vi "Queue Byte.vi"(8 "error in":errorcluster, 10 "byte":u8 format="%02x", 11 "Buffer":refnum<data-value>) -> (0 "error out":errorcluster, 1 "overflowed?":bool, 2 "overflow":u8 format="%02x", 3 "Buffer":refnum<data-value>)   [LabVIEW 2013, in "CircularBuffer.lvlib" / "ByteFIFO.lvclass"]
doc: "This VI writes one data element into the current location in the buffer. The location in the buffer is updated automatically."
uses:
  ByteFIFO.lvclass
  VariantBuffer/VariantBuffer.lvclass
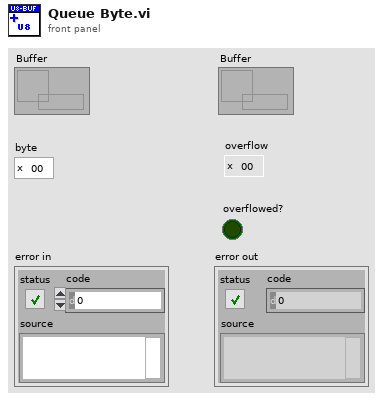
[diagram p1: front panel]
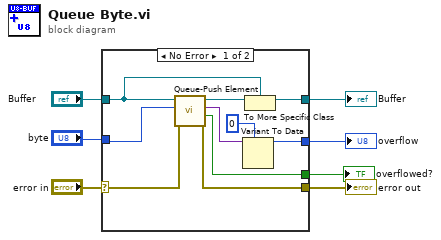
[diagram p0: block diagram]
diagram:
  n1 = case shown="No Error" "error in" {
    selector: "error in" -> [w15 w19]
    tunnel: "Buffer" -> [w12 w18]
    tunnel: [w13 w18] -> w6
    tunnel: [w14 w19] -> w5
    tunnel: "byte" -> [w17 _]
    tunnel: [w10 _] -> w2
    tunnel: [w9 _] -> w1
    frame No Error {
      n2 = call "Queue-Push Element.vi"("error in"=w15, "element"=w17, "Buffer in"=w12) -> ("error out"=w14:errorcluster, "overflowed"=w9:bool, "overflow"=w11:variant, "Buffer"=w16:refnum<data-value>)  [unwired: 5 in]
      n3 = Variant To Data(type=u8 0, Variant=w11) -> (data=w10:u8)  [unwired: 1 in, 1 out]
      n4 = To More Specific Class(target class=w12, reference=w16) -> (specific class reference=w13:refnum<data-value>)  [unwired: 1 in, 1 out]
    }
    frame Error {
    }
  }
  "error out" <- w5
  "Buffer" <- w6
  "overflow" <- w2
  "overflowed?" <- w1
